vi "Get_Data.vi"(8 "error in (no error)":errorcluster caption="entrée d'erreur (pas d'erreur)", 11 "Firebase Benches en entrée":refnum<class "Firebase Benches P2193.lvclass">) -> (0 "error out":errorcluster caption="sortie d'erreur", 3 "Firebase Benches en sortie":refnum<class "Firebase Benches P2193.lvclass">)   [LabVIEW 2020, in "Library Instrument & Equipement.lvlib" / "Library FireBase.lvlib" / "Firebase Benches P2193.lvclass"]
doc: "Returns all data Use Nb_To_Read to determine the number to read\nPlease initialise the following values\n - Name BDD\n - Document\n - API Key\n - Nb To Read"
uses:
  Firebase Benches P2193.lvclass
  C:/Users/ngarcin/OneDrive - Altyor/Standard TB/Class/Firebase/Source/Firebase Altyor/Firebase Altyor.lvclass
  C:/Users/ngarcin/OneDrive - Altyor/Standard TB/Class/Firebase/Source/Firebase Driver/Firebase Driver.lvclass
  Firebase Benches P2193.lvclass/Firebase Benches P2193.ctl
  JSON API/JSON Value/Set from JSON string.vi
  JSON API/JSON Value/JSON Value.lvclass
  Firebase Altyor/Firebase Altyor.lvclass
  JSON API/Variant JSON/Variant JSON.lvlib
  JSON API/Get Polymorphic/JSON GetSet.lvlib
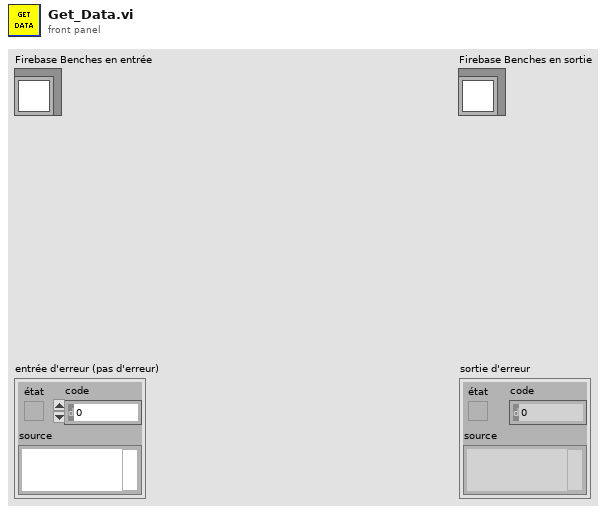
[diagram p1: front panel]
types:
  T1 = cluster{"name":string, "fields":cluster{"Result":cluster{"booleanValue":bool}, "CreationDate":cluster{"timestampValue":string}, "Batch":cluster{"stringValue":string}, "SerialNumber":cluster{"stringValue":string}, "EndOfProduction":cluster{"timestampValue":string}, "FW_Version":cluster{"mapValue":cluster{"fields":cluster{"Bootloader":cluster{"mapValue":cluster{"fields":cluster{"File_Name":cluster{"stringValue":string}, "Version":cluster{"mapValue":cluster{"fields":cluster{"Major":cluster{"stringValue":string}, "Minor":cluster{"stringValue":string}}}}, "Checksum":cluster{"stringValue":string}}}}, "SoftDevice":cluster{"mapValue":cluster{"fields":cluster{"File_Name":cluster{"stringValue":string}, "Version":cluster{"mapValue":cluster{"fields":cluster{"Major":cluster{"stringValue":string}, "Minor":cluster{"stringValue":string}}}}, "Checksum":cluster{"stringValue":string}}}}, "DFU":cluster{"mapValue":cluster{"fields":cluster{"File_Name":cluster{"stringValue":string}, "Version":cluster{"mapValue":cluster{"fields":cluster{"Major":cluster{"stringValue":string}, "Minor":cluster{"stringValue":string}}}}, "Checksum":cluster{"stringValue":string}}}}}}}, "PartNumber":cluster{"stringValue":string}, "OrderNumber":cluster{"stringValue":string}, "Operator":cluster{"stringValue":string}, "SN_CPU":cluster{"stringValue":string}}}[]
  T2 = cluster{"documents":cluster{"name":string, "fields":cluster{"Result":cluster{"booleanValue":bool}, "CreationDate":cluster{"timestampValue":string}, "Batch":cluster{"stringValue":string}, "SerialNumber":cluster{"stringValue":string}, "EndOfProduction":cluster{"timestampValue":string}, "FW_Version":cluster{"mapValue":cluster{"fields":cluster{"Bootloader":cluster{"mapValue":cluster{"fields":cluster{"File_Name":cluster{"stringValue":string}, "Version":cluster{"mapValue":cluster{"fields":cluster{"Major":cluster{"stringValue":string}, "Minor":cluster{"stringValue":string}}}}, "Checksum":cluster{"stringValue":string}}}}, "SoftDevice":cluster{"mapValue":cluster{"fields":cluster{"File_Name":cluster{"stringValue":string}, "Version":cluster{"mapValue":cluster{"fields":cluster{"Major":cluster{"stringValue":string}, "Minor":cluster{"stringValue":string}}}}, "Checksum":cluster{"stringValue":string}}}}, "DFU":cluster{"mapValue":cluster{"fields":cluster{"File_Name":cluster{"stringValue":string}, "Version":cluster{"mapValue":cluster{"fields":cluster{"Major":cluster{"stringValue":string}, "Minor":cluster{"stringValue":string}}}}, "Checksum":cluster{"stringValue":string}}}}}}}, "PartNumber":cluster{"stringValue":string}, "OrderNumber":cluster{"stringValue":string}, "Operator":cluster{"stringValue":string}, "SN_CPU":cluster{"stringValue":string}}}[], "nextPageToken":string}
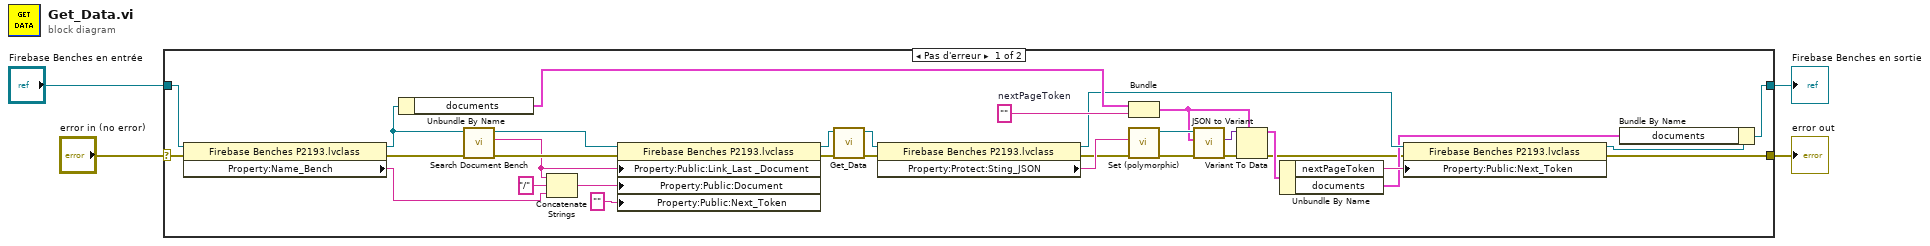
[diagram p0: block diagram]
diagram:
  n1 = case shown="Pas d'erreur" "error in (no error)" {
    selector: "error in (no error)" -> [w8 w38]
    tunnel: [w17 w37] -> w4
    tunnel: "Firebase Benches en entrée" -> [w10 w37]
    tunnel: [w14 w38] -> w2
    frame No Error {
      w26 = ""  # nextPageToken
      n2 = property class="Firebase Benches P2193.lvclass"(reference=w10, error in=w8) -> (reference out=w9:refnum<class "Firebase Benches P2193.lvclass">, error out=w7:errorcluster, "Property:Name_Bench"=w6:string)
      n3 = Unbundle By Name(w9) -> ("documents"=w25:T1)
      n4 = call "Search Document Bench.vi"("entrée d'erreur (pas d'erreur)"=w7, "Firebase Altyor en entrée"=w9) -> ("sortie d'erreur"=w13:errorcluster, "Source"=w11:string, "Firebase Altyor en sortie"=w12:refnum<class "Firebase Benches P2193.lvclass">)  [unwired: 7 in]
      n5 = Concatenate Strings(w11, "/" ("chaîne"), w6) -> (w36:string)
      n6 = property class="Firebase Benches P2193.lvclass"(reference=w12, error in=w13, "Property:Public:Link_Last _Document"=w11, "Property:Public:Document"=w36, "Property:Public:Next_Token"="" ("Next_Token")) -> (reference out=w33:refnum<class "Firebase Benches P2193.lvclass">, error out=w32:errorcluster)
      n7 = call-parent "Get_Data.vi"("error in (no error)"=w32, "Firebase Altyor en entrée"=w33) -> ("error out"=w19:errorcluster, "Firebase Altyor en sortie"=w18:refnum<class "Firebase Benches P2193.lvclass">)  [unwired: 8 in]
      n8 = property class="Firebase Benches P2193.lvclass"(reference=w18, error in=w19) -> (reference out=w23:refnum<class "Firebase Benches P2193.lvclass">, error out=w16:errorcluster, "Property:Protect:Sting_JSON"=w28:string)
      n9 = Bundle("documents"=w25, "nextPageToken"=w26) -> (w24:T2)  [unwired: 1 in]
      n10 = call-poly "Set (polymorphic).vi"("error in (no error)"=w16, "JSON stream"=w28) -> ("error out"=w29:errorcluster, "JSON Value out"=w31:refnum<class "JSON Value.lvclass">)  [unwired: 7 in, 1 out]
      n11 = call "JSON to Variant.vi"("error in (no error)"=w29, "Variant (Data Type)"=w24, "JSON Value"=w31) -> ("error out"=w30:errorcluster, "Variant out"=w5:variant)  [unwired: 7 in]
      n12 = Variant To Data(error in=w30, type=w24, Variant=w5) -> (data=w27:T2, error out=w15:errorcluster)
      n13 = Unbundle By Name(w27) -> ("nextPageToken"=w22:string, "documents"=w20:T1)
      n14 = property class="Firebase Benches P2193.lvclass"(reference=w23, error in=w15, "Property:Public:Next_Token"=w22) -> (reference out=w21:refnum<class "Firebase Benches P2193.lvclass">, error out=w14:errorcluster)
      n15 = Bundle By Name(cluster=w21, "documents"=w20) -> (w17:refnum<class "Firebase Benches P2193.lvclass">)
    }
    frame Error {
    }
  }
  "Firebase Benches en sortie" <- w4
  "error out" <- w2
